vi "Get Test Limits.vi"(4 "Position":u32, 6 "Write Limits (True)":bool=TRUE, 8 "error in (no error)":errorcluster, 10 "Channel":string, 11 "Test Class in":refnum<class "Test Class.lvclass">) -> (0 "error out":errorcluster, 2 "Lower Limit":dbl, 3 "Upper Limit":dbl)   [LabVIEW 2015, in "Test Class.lvclass"]
uses:
  Test Class.lvclass
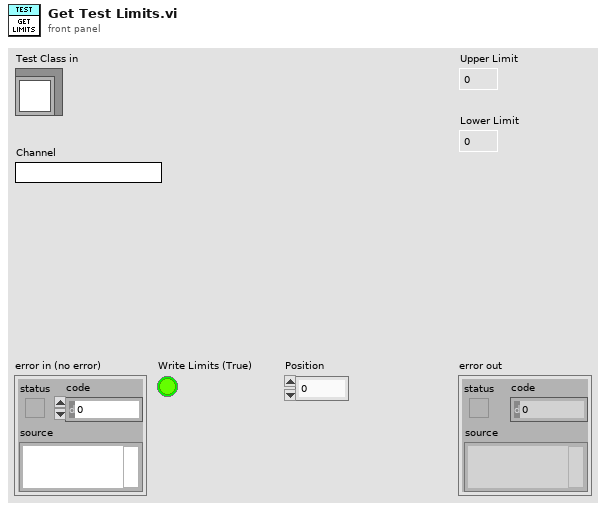
[diagram p1: front panel]
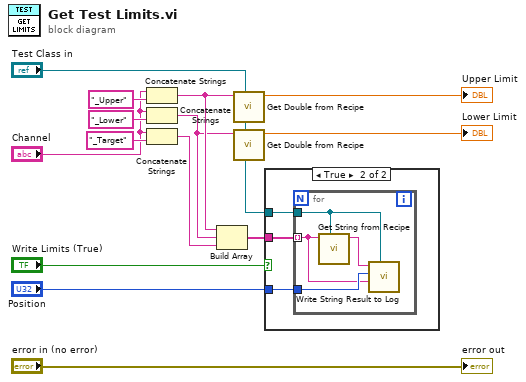
[diagram p0: block diagram]
diagram:
  n1 = Concatenate Strings("Channel", "_Upper" ("string")) -> (w5:string)
  n2 = Concatenate Strings("Channel", "_Lower" ("string")) -> (w4:string)
  n3 = Concatenate Strings("Channel", "_Target" ("string")) -> (w6:string)
  n4 = Build Array(w5, w4, w6) -> (w13:string[])
  n5 = call "Get Double from Recipe.vi"("Test Class in"="Test Class in", "Name"=w5) -> ("Value"=→"Upper Limit":dbl)  [unwired: 7 in, 2 out]
  n6 = call "Get Double from Recipe.vi"("Test Class in"="Test Class in", "Name"=w4) -> ("Value"=→"Lower Limit":dbl)  [unwired: 7 in, 2 out]
  n7 = case shown="True" "Write Limits (True)" {
    tunnel: w13 -> [_ w17]
    tunnel: "Position" -> [_ w16]
    tunnel: "Test Class in" -> [_ w15]
    frame False {
    }
    frame True {
      n8 = for {
        tunnel: w17 -> [w18] mode=indexing
        tunnel: w16 -> [w20]
        tunnel: w15 -> [w21]
        n9 = call "Get String from Recipe.vi"("Test Class in"=w21, "Name"=w18) -> ("Value"=w19:string)  [unwired: 7 in, 2 out]
        n10 = call "Write String Result to Log.vi"("Test Class in"=w21, "Label"=w18, "Position"=w20, "Value"=w19) -> ()  [unwired: 7 in, 1 out]
      }
    }
  }
  "error out" <- "error in (no error)"
